vi "UMB_UnderCloud.vi"(8 "behavior weights":i8[](array[numeric]), 11 "Boat Heading":i32) -> (3 "Behavior Output":T1)   [LabVIEW 2012]
uses:
  NINJA Code/Tugboat/Robo_Programs/behaviorOutput_t.ctl
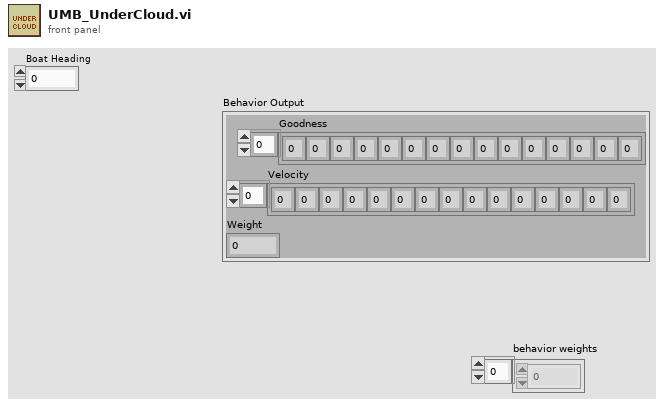
[diagram p1: front panel]
types:
  T1 = typedef "behaviorOutput_t.ctl" = cluster{"Goodness":i8[], "Velocity":i8[], "Weight":i8}
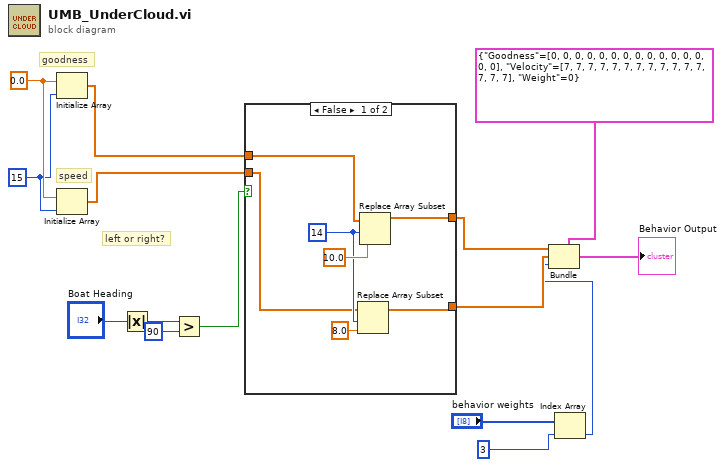
[diagram p0: block diagram]
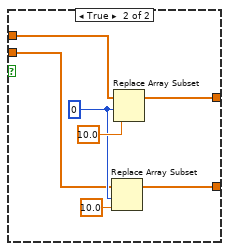
[diagram p2: hidden frame]
diagram:
  w14 = 15 ("dimension size")
  w15 = 0.0 ("element")
  # "left or right?"
  # "goodness"
  # "speed"
  n1 = Initialize Array(w15, w14) -> (w9:dbl[])
  n2 = Initialize Array(w15, w14) -> (w8:dbl[])
  n3 = Absolute Value(x="Boat Heading") -> (abs(x)=w12:i32)
  n4 = Greater?(x=w12, y=90) -> (0:w10:bool)
  n5 = case shown="False" w10 {
    tunnel: w9 -> [w19 w28]
    tunnel: w8 -> [w18 w24]
    tunnel: [w16 w27] -> w4
    tunnel: [w17 w23] -> w5
    frame False {
      w21 = 14 ("index")
      n6 = Replace Array Subset(array=w18, new element=8.0 ("new element/subarray"), index=w21) -> (w17:dbl[])
      n7 = Replace Array Subset(array=w19, new element=10.0 ("new element/subarray"), index=w21) -> (w16:dbl[])
    }
    frame True {
      w26 = 0 ("index")
      n8 = Replace Array Subset(array=w24, new element=10.0 ("new element/subarray"), index=w26) -> (w23:dbl[])
      n9 = Replace Array Subset(array=w28, new element=10.0 ("new element/subarray"), index=w26) -> (w27:dbl[])
    }
  }
  n10 = Index Array(array="behavior weights", index=3) -> (element=w1:i8)
  n11 = Bundle(cluster=T1 {"Goodness"=[0, 0, 0, 0, 0, 0, 0, 0, 0, 0, 0, 0, 0, 0, 0], "Velocity"=[7, 7, 7, 7, 7, 7, 7, 7, 7, 7, 7, 7, 7, 7, 7], "Weight"=0} ("Behavior Output"), "Goodness"=w4, "Velocity"=w5, "Weight"=w1) -> (→"Behavior Output":T1)
